vi "Get_Spec_Wavelength.vi"(8 "error in (no error)":errorcluster, 11 ".NET Reference in":refnum<k24>) -> (0 "error out":errorcluster, 1 "minwave":dbl, 2 "maxwave":dbl, 3 "Reference out":refnum<k24>)   [LabVIEW 2017]
doc: "Add the spec wavelength to Dictionary"
uses:
  LV_IL_Sample/DLL/InstrumentDLL.dll
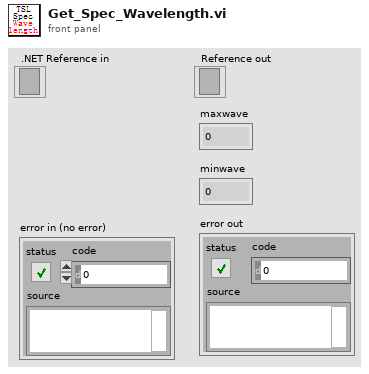
[diagram p1: front panel]
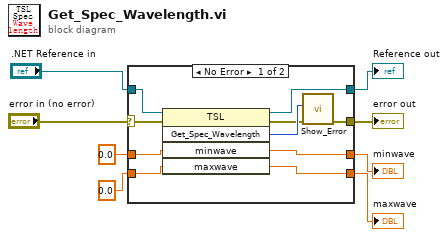
[diagram p0: block diagram]
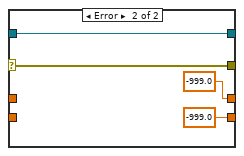
[diagram p2: hidden frame]
diagram:
  n1 = case shown="No Error" "error in (no error)" {
    selector: "error in (no error)" -> [w9 w22]
    tunnel: ".NET Reference in" -> [w18 w21]
    tunnel: [w17 w21] -> w7
    tunnel: [w10 w22] -> w6
    tunnel: 0.0 ("minwave") -> [w16 _]
    tunnel: 0.0 ("maxwave") -> [w15 _]
    tunnel: [w14 -999.0 ("minwave")] -> w3
    tunnel: [w13 -999.0 ("maxwave")] -> w2
    frame No Error {
      n2 = invoke on="调用节点" class="TSL" method="Get_Spec_Wavelength"(reference=w18, error in=w9, "minwave"=w16, "maxwave"=w15) -> (reference out=w17:refnum<k24>, error out=w11:errorcluster, "Get_Spec_Wavelength"=w12:i32, "minwave"=w14:dbl, "maxwave"=w13:dbl)  [unwired: 1 in]
      n3 = call "Show_Error.vi"("error in (no error)"=w11, "Error"=w12) -> ("error out"=w10:errorcluster)  [unwired: 9 in]
    }
    frame Error {
    }
  }
  "Reference out" <- w7
  "error out" <- w6
  "minwave" <- w3
  "maxwave" <- w2
